vi "get_logic_statement_statuses.vi"(8 "error in (no error)":errorcluster, 11 "VISA resource name":refnum<visa-resource-name>) -> (0 "error out":errorcluster, 2 "logic statement status array":bool[](array[boolean]), 3 "VISA resource name out":refnum<visa-resource-name>)   [LabVIEW 2018]
doc: "Read the status of all logic statements."
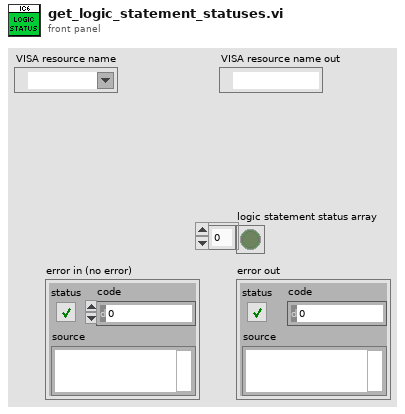
[diagram p1: front panel]
types:
  T1 = enum16{"Source", "General", "Input name", "Process name", "Logic", "Material", "Material name", "Output name", "Process", "Sensor", "Output type", "User message", "Layer", ""}
  T2 = enum16{"Hello", "Query", "Remote action", "Status", "Update"}
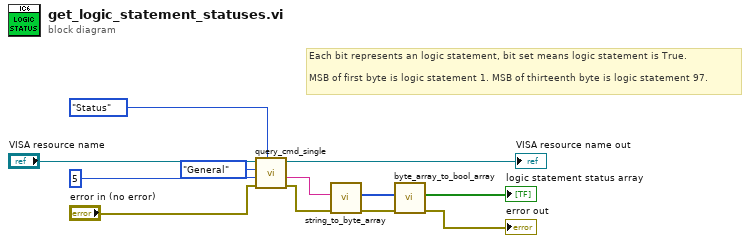
[diagram p0: block diagram]
diagram:
  # "Each bit represents an logic statement, bit set means logic statement is True. \n\nMSB of first byte is logic statement 1. MSB of thirteenth byte is logic statement 97."
  n1 = call "query_cmd_single.vi"("Command group"=T2."Status", "error in (no error)"="error in (no error)", "Command ID"=u8 5, "Command subgroup"=T1."General", "VISA resource name"="VISA resource name") -> ("error out"=w7:errorcluster, "formatted response"=w2:string, "VISA resource name out"=→"VISA resource name out":refnum<visa-resource-name>)  [unwired: 2 in, 2 out]
  n2 = call "string_to_byte_array.vi"("error in (no error)"=w7, "Byte"=w2) -> ("error out"=w6:errorcluster, "Int array"=w3:u8[])  [unwired: 8 in]
  n3 = call "byte_array_to_bool_array.vi"("error in (no error)"=w6, "Byte array"=w3) -> ("error out"=→"error out":errorcluster, "Boolean array"=→"logic statement status array":bool[])  [unwired: 8 in]
